vi "Prober_MoveToHome.vi"(8 "error in (no error)":errorcluster, 11 "TeslaVeloxProbeStation in":refnum<class "TeslaVeloxProbeStation.lvclass">) -> (0 "error out":errorcluster, 3 "TeslaVeloxProbeStation out":refnum<class "TeslaVeloxProbeStation.lvclass">)   [LabVIEW 2018, in "TeslaVeloxProbeStation.lvclass"]
uses:
  TeslaVeloxProbeStation.lvclass
  Desktop/Kvasnicka/test_labview_library/Integration_toolkit_library/CascadeProbestation.lvlib
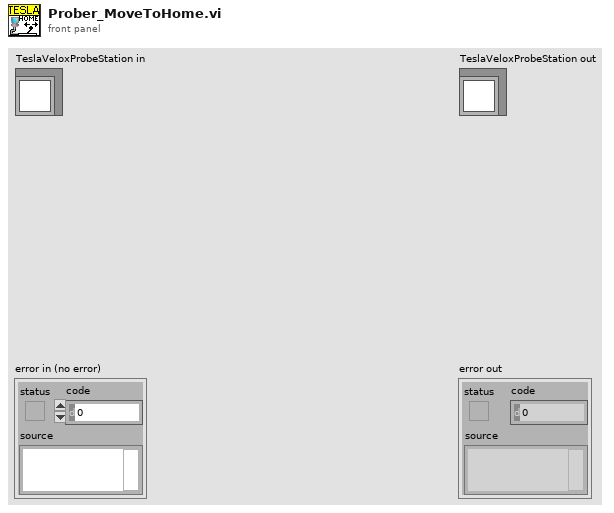
[diagram p1: front panel]
types:
  T1 = enum16{"Home", "Zero", "Center", "Current position"}
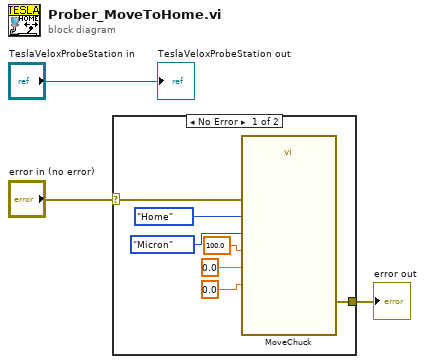
[diagram p0: block diagram]
diagram:
  n1 = case shown="No Error" "error in (no error)" {
    selector: "error in (no error)" -> [w9 w11]
    tunnel: [w10 w11] -> w2
    frame No Error {
      n2 = call "MoveChuck.vi"("X Value"=0.0, "Velocity"=100.0, "Y Value"=0.0, "PosRef"=T1."Home", "Unit"=enum16{"Micron", "Mils", "Index", "Jog"}."Micron", "Error In"=w9) -> ("Error Out"=w10:errorcluster)  [unwired: 8 in, 1 out]
    }
    frame Error {
    }
  }
  "error out" <- w2
  "TeslaVeloxProbeStation out" <- "TeslaVeloxProbeStation in"
